vi "Launch Write Request Spawn.vi"(8 "error in (no error)":errorcluster, 9 "Caller Return Queue":refnum<queue>, 10 "Request Queue":refnum<queue>, 11 "Number of Requests":i32) -> (0 "error out":errorcluster)   [LabVIEW 2017, in "Network Interface.lvlib" / "Network Session Handler.lvclass"]
uses:
  <vilib>/gpm_packages/@cs/Network-sink/Source/Network Interface/Network Session Handler/Network Session Handler.lvclass
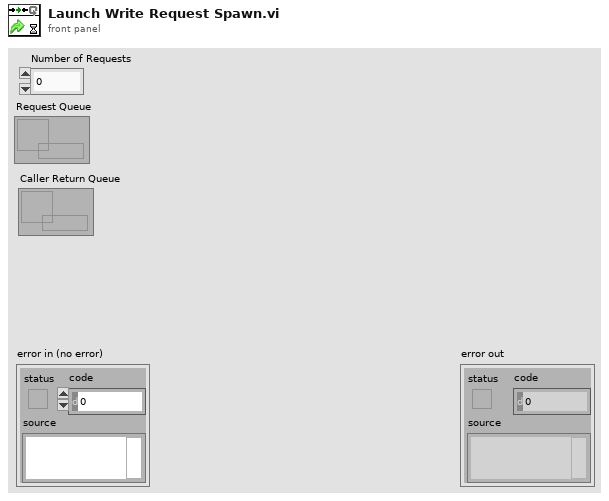
[diagram p1: front panel]
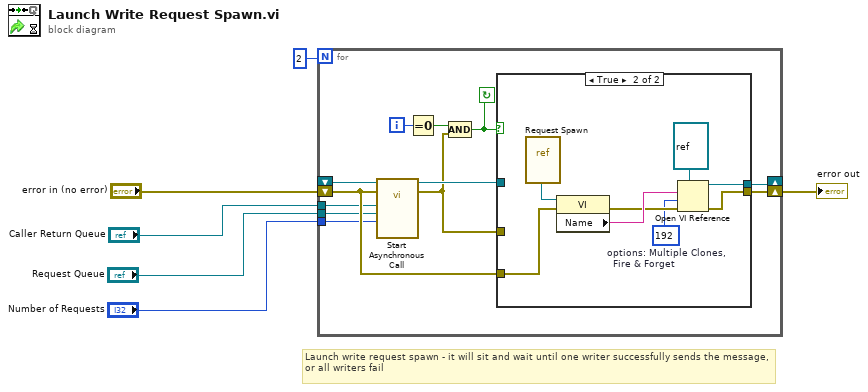
[diagram p0: block diagram]
diagram:
  # "Launch write request spawn - it will sit and wait until one writer successfully sends the message, or all writers fail"
  n1 = for {
    N: 2 -> [_]
    shift-right: [w17] -> _
    shift-left: _ -> [w18]
    shift-right: [w12] -> w2
    shift-left: "error in (no error)" -> [w11]
    tunnel: "Caller Return Queue" -> [w9]
    tunnel: "Request Queue" -> [w8]
    tunnel: "Number of Requests" -> [w7]
    i -> [w14]
    stop <- w10 continue-if-true
    n2 = call-by-ref "Start Asynchronous Call"(reference=w18, error in=w11, "Number of Requests"=w7, "Request Queue"=w8, "Return Queue"=w9) -> (reference out=w16:refnum<vi>, error out=w13:errorcluster)  [unwired: 9 in]
    n3 = Equal To 0?(x=w14) -> (x = 0?=w15:bool)
    n4 = Compound Arithmetic op=AND(w15, w13) -> (w10:bool)
    n5 = case shown="True" w10 {
      tunnel: [w20 w25] -> w17
      tunnel: w16 -> [w20 _]
      tunnel: w13 -> [w19 _]
      tunnel: [w19 w23] -> w12
      tunnel: w11 -> [_ w22]
      frame False {
      }
      frame True {
        w21 = 192  # options: Multiple Clones,   Fire & Forget
        n6 = vi-ref <vilib>:"Request Spawn.vi"() -> (w28:refnum<vi>)
        n7 = property class="VI"(reference=w28, error in=w22) -> (error out=w24:errorcluster, "Name"=w27:string)  [unwired: 1 out]
        n8 = Open VI Reference(type specifier VI Refnum (for type only)=refnum<vi> refnum, vi path=w27, options=w21, error in (no error)=w24) -> (vi reference=w25:refnum<vi>, error out=w23:errorcluster)  [unwired: 2 in]
      }
    }
  }
  "error out" <- w2
